vi "Triangle Wave Start.vi"() -> ()   [LabVIEW 2014]
panel:
  out "String":string="Triangle Wave Generator\n\nDO NOT CLOSE IF YOU WANT TO USE THE \nQ-METER"
  in  "stop (F)":bool
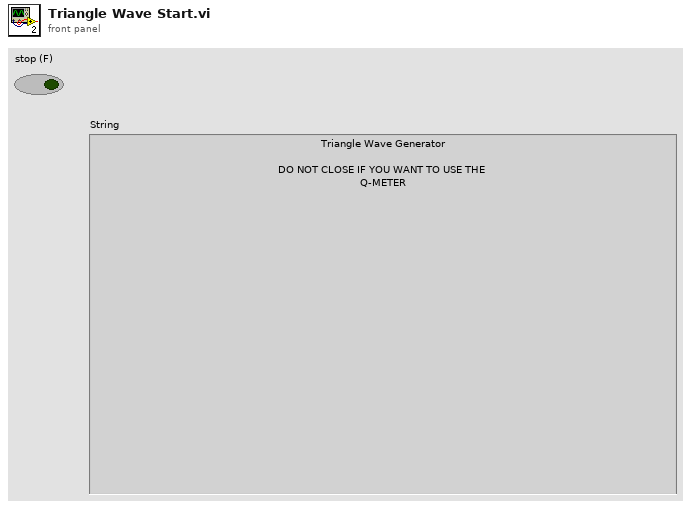
[diagram p1: front panel]
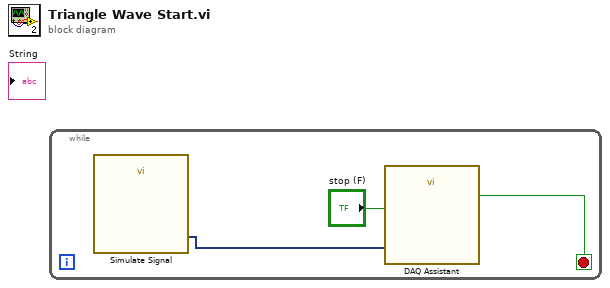
[diagram p0: block diagram]
diagram:
  n1 = while {
    stop <- w2 stop-if-true
    n2 = call "Simulate Signal"() -> ("Triangle"=w1:dynamicdata)  [unwired: 14 in, 1 out]
    n3 = call "DAQ Assistant"("data"=w1, "stop (F)"="stop (F)") -> ("stopped"=w2:bool)  [unwired: 15 in, 2 out]
  }
